vi "Waveform data class VI - retrieve FFT data.vi"(0 "Waveform data in":refnum<class "Waveform data.lvclass">, 11 "error in (no error)":errorcluster) -> (4 "Waveform data out":refnum<class "Waveform data.lvclass">, 6 "Angles FFT":dbl[](array[numeric]), 8 "displacement FFT":dbl[](array[numeric]), 15 "error out":errorcluster)   [LabVIEW 2010, in "Waveform data.lvclass"]
uses:
  Waveform data.lvclass
  Waveform data.lvclass/Waveform data.ctl
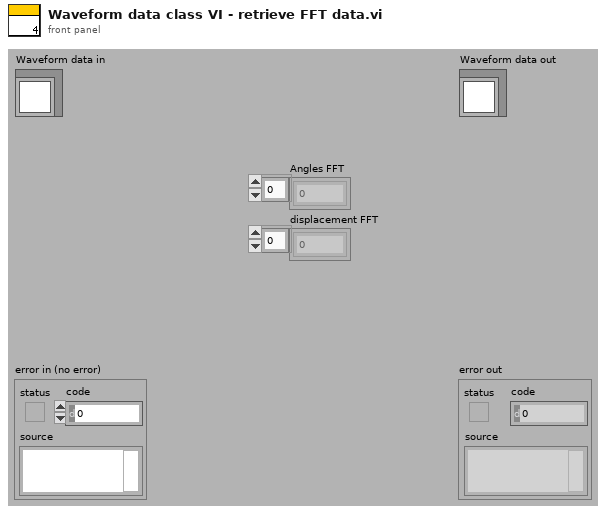
[diagram p1: front panel]
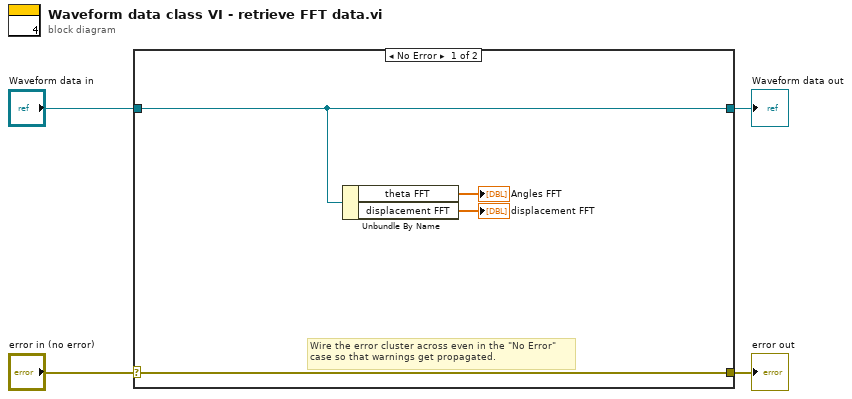
[diagram p0: block diagram]
diagram:
  n1 = case shown="No Error" "error in (no error)" {
    selector: "error in (no error)" -> [w8 w10]
    tunnel: [w8 w10] -> w3
    tunnel: [w7 w9] -> w1
    tunnel: "Waveform data in" -> [w7 w9]
    frame No Error {
      # "Wire the error cluster across even in the \"No Error\"\ncase so that warnings get propagated."
      n2 = Unbundle By Name(w7) -> ("theta FFT"=→"Angles FFT":dbl[], "displacement FFT"=→"displacement FFT":dbl[])
    }
    frame Error {
    }
  }
  "error out" <- w3
  "Waveform data out" <- w1
